vi "MIMIC Globals.vi"() -> ()   [LabVIEW 2014]
panel:
  in  "G_MIMIC_HOST_PORT":refnum<visa-resource-name>
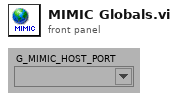
[diagram p1: front panel]
diagram:
